vi "CMD_CLEARVARS.vi"(8 "error in (no error)":errorcluster, 10 "Arguments":string[](array[string]), 11 "gScript Interpreter in":refnum<class "gScript Interpreter.lvclass">) -> (0 "error out":errorcluster, 3 "gScript Interpreter out":refnum<class "gScript Interpreter.lvclass">)   [LabVIEW 2023, in "gScript Interpreter.lvclass"]
uses:
  gScript Interpreter.lvclass
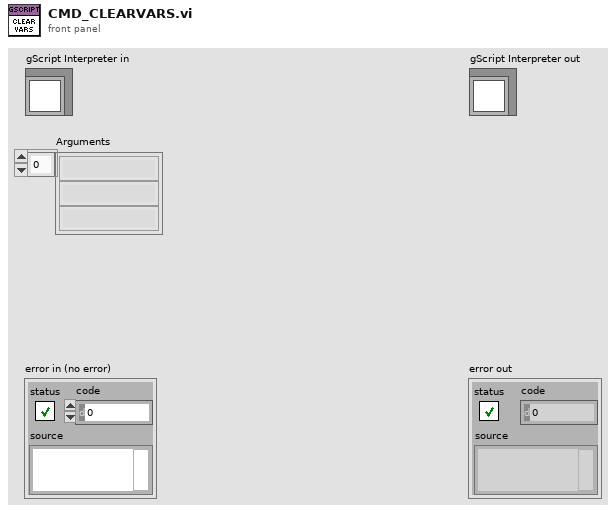
[diagram p1: front panel]
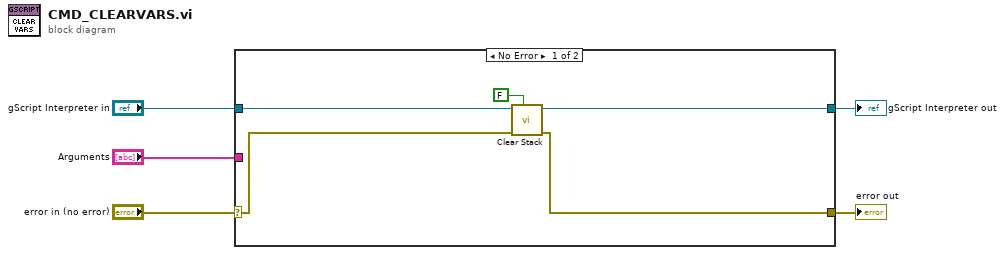
[diagram p0: block diagram]
diagram:
  n1 = case shown="No Error" "error in (no error)" {
    selector: "error in (no error)" -> [w8 w12]
    tunnel: [w7 w12] -> w4
    tunnel: [w6 w11] -> w2
    tunnel: "gScript Interpreter in" -> [w10 w11]
    tunnel: "Arguments" -> [_ _]
    frame No Error {
      n2 = call "Clear Stack.vi"("Keep Base Frame"=FALSE, "error in (no error)"=w8, "gScript Interpreter in"=w10) -> ("error out"=w7:errorcluster, "gScript Interpreter out"=w6:refnum<class "gScript Interpreter.lvclass">)  [unwired: 7 in]
    }
    frame Error {
    }
  }
  "error out" <- w4
  "gScript Interpreter out" <- w2
